vi "SPD.HV_Bias Build Grid.vi"(6 "min delta V":dbl, 8 "error in (no error)":errorcluster, 9 "Num Of intervals":i32, 10 "HV_bias min":dbl, 11 "HV_bias max":dbl) -> (0 "error out":errorcluster, 1 "wait before next meas":bool, 2 "HV_bias Grid":dbl[](array[numeric]))   [LabVIEW 2018]
uses:
  <vilib>/Analysis/1siggen.llb/Ramp Pattern by Samples.vi
  <vilib>/Utility/error.llb/Error Cluster From Error Code.vi
  <vilib>/ErrorRing/Error Ring.xnode
  <vilib>/Analysis/NI_AALBase.lvlib
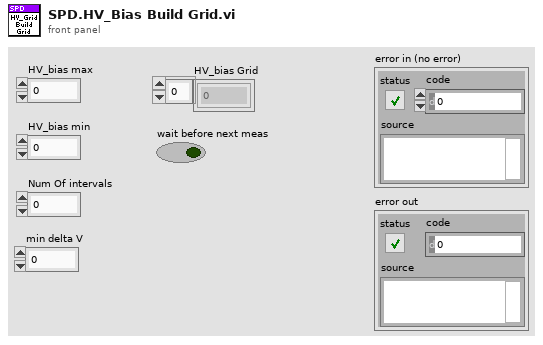
[diagram p1: front panel]
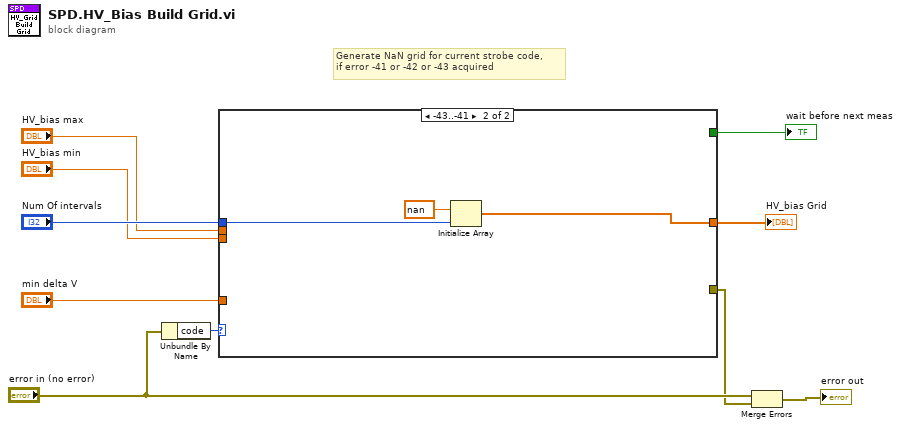
[diagram p0: block diagram]
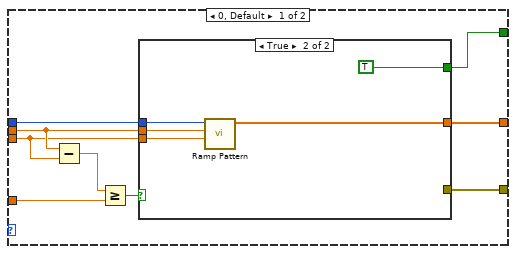
[diagram p2: hidden frame]
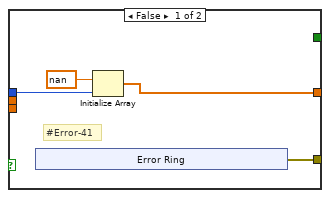
[diagram p3: hidden frame]
diagram:
  # "Generate NaN grid for current strobe code, \nif error -41 or -42 or -43 acquired"
  n1 = Unbundle By Name("error in (no error)") -> ("code"=w9:i32)
  n2 = case shown="-43..-41" w9 {
    tunnel: [w19 w34] -> w5
    tunnel: "HV_bias max" -> [w17 _]
    tunnel: "HV_bias min" -> [w16 _]
    tunnel: "Num Of intervals" -> [w18 w36]
    tunnel: [w11 _] -> w10
    tunnel: "min delta V" -> [w14 _]
    tunnel: [w12 _] -> w1
    frame 0, Default {
      n3 = Subtract(x=w17, y=w16) -> (x-y=w15:dbl)
      n4 = Greater Or Equal?(x=w15, y=w14) -> (x >= y?=w13:bool)
      n5 = case shown="True" w13 {
        tunnel: [w21 w33] -> w19
        tunnel: w18 -> [w22 w32]
        tunnel: w17 -> [_ w31]
        tunnel: w16 -> [_ w30]
        tunnel: [w20 _] -> w12
        tunnel: [_ TRUE] -> w11
        frame False {
          # "#Error-41"
          n6 = xnode "Error Ring"() -> ("error out"=w20:errorcluster)
          n7 = Initialize Array(nan ("element"), w22) -> (w21:dbl[])
        }
        frame True {
          n8 = call-poly <vilib>:"Ramp Pattern.vi"("start"=w30, "end"=w31, "samples"=w32) -> ("Ramp Pattern"=w33:dbl[])  [unwired: 7 in, 1 out]
        }
      }
    }
    frame -43..-41 {
      n9 = Initialize Array(nan ("element"), w36) -> (w34:dbl[])
    }
  }
  "wait before next meas" <- w10
  "HV_bias Grid" <- w5
  n10 = Merge Errors("error in (no error)", w1) -> (→"error out":errorcluster)
